vi "GetFlattenedString.vi"(8 "error in":errorcluster, 11 "Decimal in":refnum<class "Decimal.lvclass">) -> (0 "error out":errorcluster, 2 "FlattenedString":string, 3 "Decimal out":refnum<class "Decimal.lvclass">)   [LabVIEW 2021, in "ProligentXMLGenerator.lvlib" / "Decimal.lvclass"]
uses:
  Decimal.lvclass
  Decimal.lvclass/Decimal.ctl
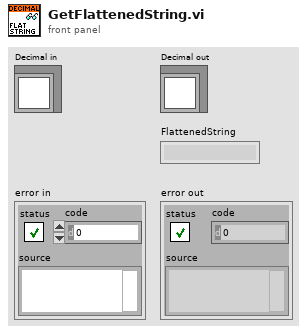
[diagram p1: front panel]
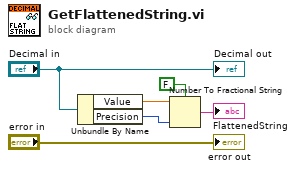
[diagram p0: block diagram]
diagram:
  n1 = Unbundle By Name("Decimal in") -> ("Value"=w3:dbl, "Precision"=w2:u8)
  n2 = Number To Fractional String(use system decimal point (T)=FALSE, number=w3, precision (6)=w2) -> (F-format string=→"FlattenedString":string)  [unwired: 1 in]
  "error out" <- "error in"
  "Decimal out" <- "Decimal in"
